vi "Display Data.vi"() -> ()   [LabVIEW 2020, in "Startup Processes.lvlib"]
uses:
  Startup Processes.lvlib
  Config Data/typedefs/Menu Context Selections.ctl
  _typedefs/Subpanel Names.ctl
  toolbox/Standard Signalling/ude_Stop Application/Get Event Reference.vi
  toolbox/Standard Signalling/ude_Stop Application/ude_Stop Application.lvlib
  toolbox/Standard Signalling/ude_Handle Errors/ude_Handle Errors.lvlib
  Dialog Boxes/Dialog Boxes.lvlib
  _ude/Change Source/Change Source.lvlib
  _buffers/Sample Rate/Sample Rate.lvlib
  _buffers/Plugin References/Plugin References.lvlib
  toolbox/User Interface/User Interface.lvlib
  Display Properties Manager/Display Properties Manager.lvlib
  Config Data/Config Data.lvclass
panel:
  in  "Menu Context":T1=enum."By Function"
  in  "Tree":string(tree)
  in  "Save Data":bool
  in  "Sample Period":i32=10000 caption="Sample Period (msec)"
  in  "stop":bool
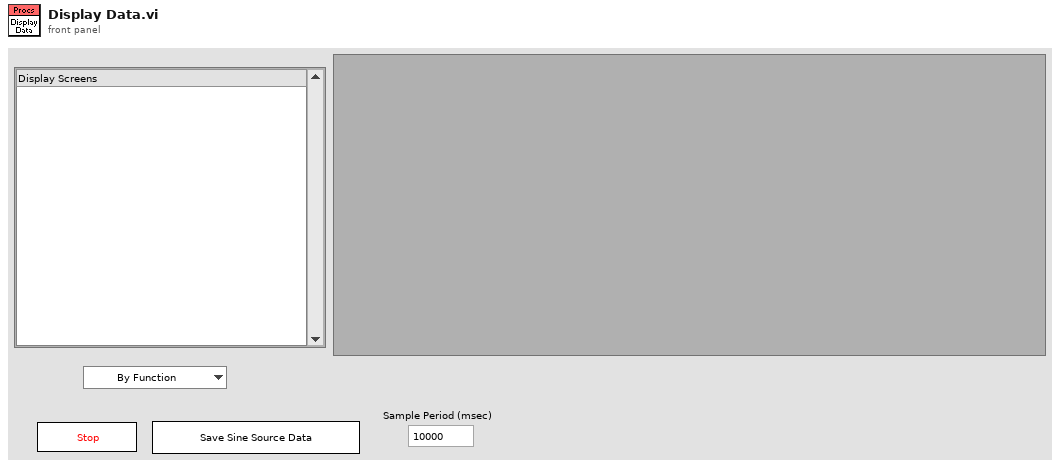
[diagram p1: front panel]
types:
  T1 = typedef "Config Data.lvlib/Config Data.lvclass/Menu Context Selections.ctl" = enum16{"By Location", "By Function"}
  T2 = typedef "Startup Processes.lvlib/Subpanel Names.ctl" = enum16{"Sine Source", "Ramp Source", "Hen House TC", "Dog House TC", "Out House TC"}
  T3 = cluster{"Source Name":T2, "Save Button":refnum<vi>, "GUI Refnum":refnum<vi>, "Menu Refnum":refnum<k9>}
  T4 = typedef "Config Data.lvlib/Config Data.lvclass/Process Launch Data.ctl" = cluster{"Label":string, "File Path":path, "Launch Mode":T5}
  T5 = typedef "Config Data.lvlib/Config Data.lvclass/Process Type.ctl" = enum16{"Async - Non-Reentrant", "Async - Reentrant", "Run Method - Non-Reentrant", "Run Method - Reentrant"}
  T6 = cluster{"Parent Tag":string, "Child Name":string, "Child Tag":string, "Child Only?":bool}[]
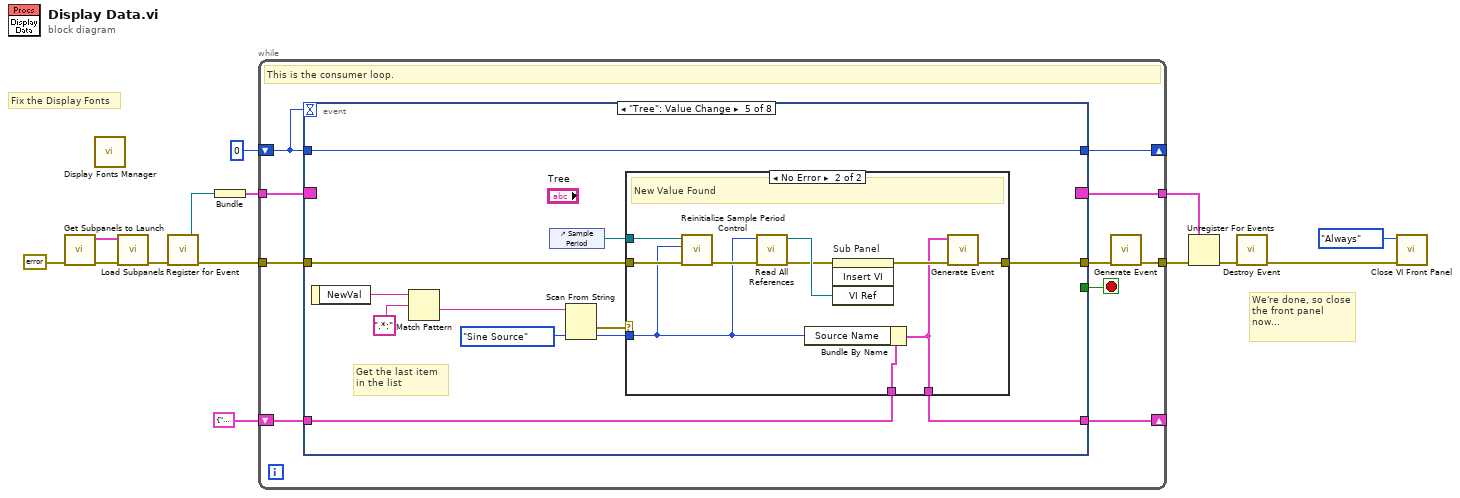
[diagram p0: block diagram]
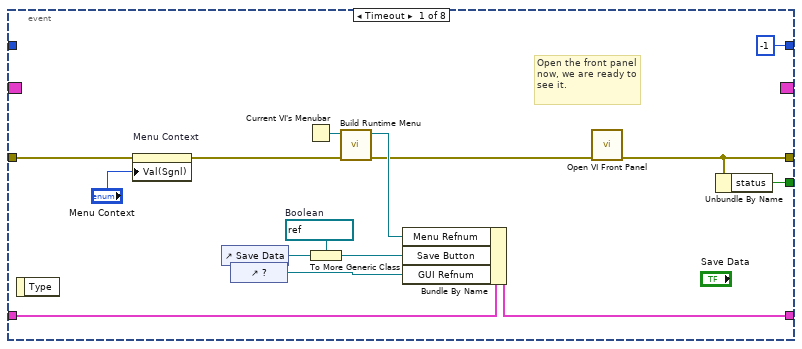
[diagram p2: hidden frame]
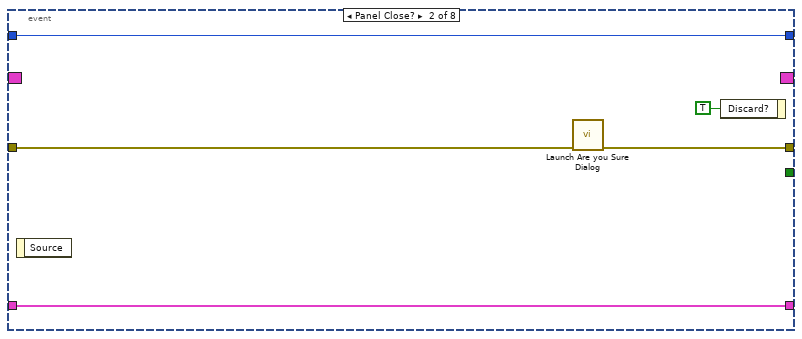
[diagram p3: hidden frame]
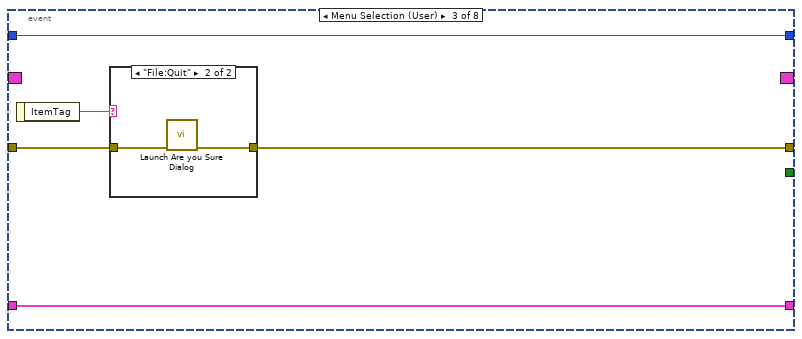
[diagram p4: hidden frame]
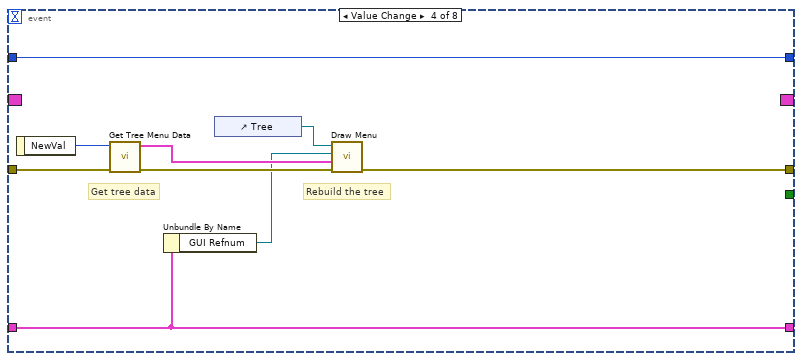
[diagram p6: hidden frame]
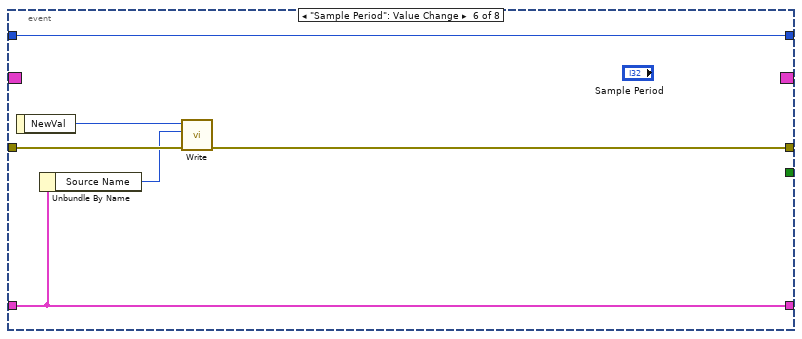
[diagram p8: hidden frame]
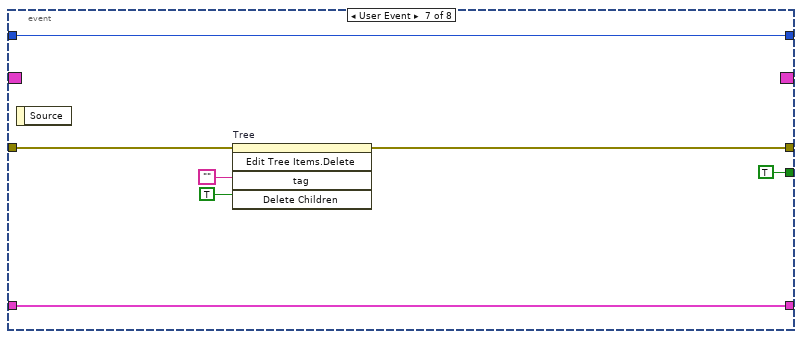
[diagram p9: hidden frame]
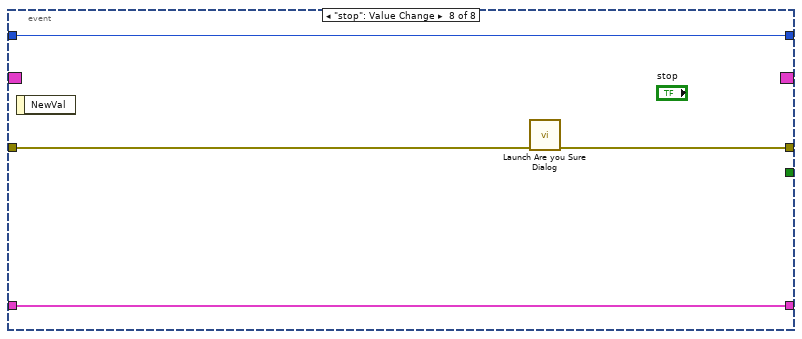
[diagram p10: hidden frame]
diagram:
  # "Fix the Display Fonts"
  # "We're done, so close the front panel now..."
  n1 = call "Get Subpanels to Launch.vi"("Error In"=errorcluster {"status"=FALSE, "code"=0, "source"=""} ("error in (no error)")) -> ("Error Out"=w2:errorcluster, "Subpanels to Launch"=w9:T4[])  [unwired: 5 in]
  n2 = call "Display Fonts Manager.vi"() -> ()  [unwired: 7 in, 1 out]
  n3 = call "Load Subpanels.vi"("error in (no error)"=w2, "Subpanels to Launch"=w9) -> ("error out"=w1:errorcluster)  [unwired: 5 in]
  n4 = call "Register for Event.vi"("Error In"=w1) -> ("Error Out"=w11:errorcluster, "sys"=w12:refnum<event-registration>)  [unwired: 5 in]
  n5 = Bundle("sys"=w12) -> (w13:cluster{"sys":refnum<event-registration>})  [unwired: 1 in]
  n6 = while {
    tunnel: w13 -> [w24]
    tunnel: w11 -> [w23]
    tunnel: [w19] -> w14
    tunnel: [w22] -> w4
    shift-right: [w18] -> _
    shift-left: 0 -> [w17]
    shift-right: [w16] -> _
    shift-left: T3 {"Source Name"=enum."Sine Source", "Save Button"=refnum, "GUI Refnum"=refnum, "Menu Refnum"=refnum} ("Event Data") -> [w15]
    stop <- w21 stop-if-true
    # "This is the consumer loop."
    n7 = event shown="[4] \"Tree\": Value Change" {
      selector: w24 -> [_ _ _ _ _ _ _ _]
      dyn-events: [_ _ _ _ _ _ _ _] -> w22
      timeout: w17 -> [_ _ _ _ _ _ _ _]
      tunnel: w23 -> [w36 w40 w46 w55 w69 w90 w95 w99]
      tunnel: [w30 w43 w45 w58 w72 w88 w94 w102] -> w20
      tunnel: [w38 _ _ _ _ _ TRUE _] -> w21
      tunnel: [-1 w42 w49 w61 w73 w89 w97 w101] -> w18
      tunnel: w17 -> [_ w42 w49 w61 w73 w89 w97 w101]
      tunnel: [w33 w41 w48 w54 w63 w87 w96 w100] -> w16
      tunnel: w15 -> [w35 w41 w48 w54 w64 w87 w96 w100]
      event Timeout {
        w28 = refnum<vi> refnum  # Boolean
        # "Open the front panel now, we are ready to see it."
        n8 = event-data() -> ()  [unwired: 1 in, 1 out]
        n9 = property on="Menu Context" class="Enum (strict)"(error in=w36, "Val(Sgnl)"="Menu Context") -> (error out=w27:errorcluster)  [unwired: 1 in, 1 out]
        n10 = control-ref of="Save Data"() -> (w31:refnum<vi>)
        n11 = control-ref of="?"() -> (w32:refnum<vi>)
        n12 = Current VI's Menubar() -> (w37:refnum<k9>)
        n13 = To More Generic Class(target class=w28, reference=w31) -> (generic class reference=w29:refnum<vi>)
        n14 = call "Build Runtime Menu.vi"("error in (no error)"=w27, "Menu in"=w37) -> ("error out"=w25:errorcluster, "Menu out"=w34:refnum<k9>)  [unwired: 4 in]
        n15 = Bundle By Name(cluster=w35, "Menu Refnum"=w34, "Save Button"=w29, "GUI Refnum"=w32) -> (w33:T3)
        n16 = call "Open VI Front Panel.vi"("error in (no error)"=w25) -> ("error out"=w30:errorcluster)  [unwired: 6 in]
        n17 = Unbundle By Name(w30) -> ("status"=w38:bool)
      }
      event Panel Close? {
        n18 = event-data() -> ()  [unwired: 1 in, 1 out]
        n19 = call "Launch Are you Sure Dialog.vi"("Error In"=w40) -> ("Error Out"=w43:errorcluster)  [unwired: 6 in]
        n20 = event-data("Discard?"=TRUE) -> ()  [unwired: 1 in, 1 out]
      }
      event Menu Selection (User) {
        n21 = event-data() -> ("ItemTag"=w47:string)  [unwired: 1 in]
        n22 = case shown="\"File:Quit\"" w47 {
          tunnel: w46 -> [w50 w52]
          tunnel: [w50 w51] -> w45
          frame Default {
          }
          frame "File:Quit" {
            n23 = call "Launch Are you Sure Dialog.vi"("Error In"=w52) -> ("Error Out"=w51:errorcluster)  [unwired: 6 in]
          }
        }
      }
      event Value Change {
        # "Rebuild the tree"
        # "Get tree data"
        n24 = event-data() -> ("NewVal"=w56:T1)  [unwired: 1 in]
        n25 = call "Get Tree Menu Data.vi"("Error In"=w55, "Menu Context"=w56) -> ("Error Out"=w60:errorcluster, "Array"=w59:T6)  [unwired: 4 in]
        n26 = Unbundle By Name(w54) -> ("GUI Refnum"=w53:refnum<vi>)
        n27 = control-ref of="Tree"() -> (w57:refnum<vi>)
        n28 = call "Draw Menu.vi"("error in (no error)"=w60, "Tree Items"=w59, "VI Reference"=w53, "TreeControl in"=w57) -> ("error out"=w58:errorcluster)  [unwired: 3 in]
      }
      event "Tree": Value Change {
        # "Get the last item in the list"
        n29 = event-data() -> ("NewVal"=w70:string)  [unwired: 1 in]
        n30 = Match Pattern(string=w70, regular expression=".*:") -> (after substring=w67:string)  [unwired: 1 in, 3 out]
        n31 = control-ref of="Sample Period"() -> (w65:refnum<vi>)
        n32 = Scan From String(input string=w67, default 1=Subpanel_Names."Sine Source" ("Plugin Names")) -> (error out=w62:errorcluster, output 1=w68:T2)  [unwired: 3 in, 2 out]
        n33 = case shown="No Error" w62 {
          tunnel: [w75 w84] -> w72
          tunnel: w64 -> [w74 w83]
          tunnel: w68 -> [_ w76]
          tunnel: w69 -> [w75 w80]
          tunnel: w65 -> [_ w78]
          tunnel: [w74 w77] -> w63
          frame Error {
            # "This case structure is to work around a bug in the tree control. Even if you have it configured to not allow parents to be selected, clicking on one will still generate a value change event, even though the value isn't really changing."
            # "Value not found"
          }
          frame No Error {
            # "New Value Found"
            n34 = call "Reinitialize Sample Period Control.vi"("error in (no error)"=w80, "Plugin Names"=w76, "Digital in"=w78) -> ("error out"=w79:errorcluster)  [unwired: 4 in]
            n35 = call "Read All References.vi"("Error In"=w79, "Plugin Names"=w76) -> ("Error Out"=w81:errorcluster, "Reference Out"=w82:refnum<vi>)  [unwired: 4 in]
            n36 = Bundle By Name(cluster=w83, "Source Name"=w76) -> (w77:T3)
            n37 = invoke on="Sub Panel" class="SubPanel" method="Insert VI"(error in=w81, "VI Ref"=w82) -> (error out=w85:errorcluster)  [unwired: 2 in, 3 out]
            n38 = call "Generate Event.vi"("Error In"=w85, "Event Data"=w77) -> ("Error Out"=w84:errorcluster)  [unwired: 5 in]
          }
        }
      }
      event "Sample Period": Value Change {
        n39 = event-data() -> ("NewVal"=w91:i32)  [unwired: 1 in]
        n40 = Unbundle By Name(w87) -> ("Source Name"=w86:T2)
        n41 = call "Write.vi"("Error In"=w90, "Plugin Name"=w86, "Sample Period (msec)"=w91) -> ("Error Out"=w88:errorcluster)  [unwired: 2 in, 2 out]
      }
      event User Event {
        n42 = event-data() -> ()  [unwired: 1 in, 1 out]
        n43 = invoke on="Tree" class="Tree (strict)" method="Edit Tree Items.Delete"(error in=w95, "tag"="", "Delete Children"=TRUE ("Delete Children?")) -> (error out=w94:errorcluster)  [unwired: 2 in, 4 out]
      }
      event "stop": Value Change {
        n44 = event-data() -> ()  [unwired: 1 in, 1 out]
        n45 = call "Launch Are you Sure Dialog.vi"("Error In"=w99) -> ("Error Out"=w102:errorcluster)  [unwired: 6 in]
      }
    }
    n46 = call "Generate Event.vi"("Error In"=w20) -> ("Error Out"=w19:errorcluster)  [unwired: 6 in]
  }
  n47 = Unregister For Events(event registration refnum=w4, error in=w14) -> (error out=w6:errorcluster)
  n48 = call "Destroy Event.vi"("Error In"=w6) -> ("Error Out"=w8:errorcluster)  [unwired: 6 in]
  n49 = call "Close VI Front Panel.vi"("Error In"=w8, "When"=enum16{"Always", "Not Development"}."Always") -> ()  [unwired: 5 in, 1 out]
